vi "ATF-Obtain Notifier.vi"(8 "error in":errorcluster) -> (0 "error out":errorcluster, 3 "Cluster":T1)   [LabVIEW 2022 SP3]
uses:
  Controls/SeCrTs-Notifier ctl.ctl
  Controls/SeCrTs-NS Data type.ctl
  Controls/Commands to log.ctl
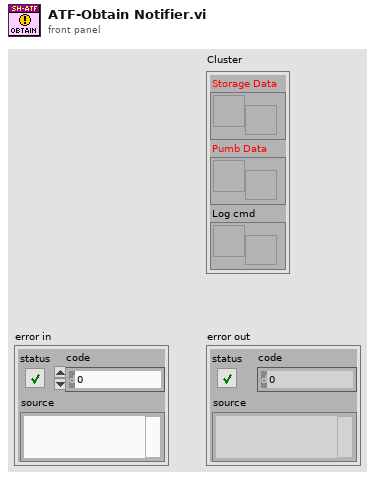
[diagram p1: front panel]
types:
  T1 = typedef "SeCrTs-Notifier ctl.ctl" = cluster{"Storage Data":refnum<notifier>, "Pumb Data":refnum<notifier>, "Log cmd":refnum<notifier>}
  T2 = typedef "Commands to log.ctl" = cluster{"C/NC":bool, "Start/Stop Log":bool[], "Log Name":string, "Config":cluster{"AO config":cluster{"Channel_Name":string, "Channel_Number":string, "Default_Value":dbl, "Units":string}[], "AI config":cluster{"Channel_Name":string, "Channel_Number":string, "Pre_Scale_min":dbl, "Pre_Scale_max":dbl, "Sensor_min":dbl, "Sensor_max":dbl, "Units":string}[], "DI config":cluster{"Channel_Name":string, "Channel_Number":string, "Default_Value":bool, "DI invert?":bool}[], "DO config":cluster{"Channel_Name":string, "Channel_Number":string, "Default_Value":bool, "DO invert?":bool}[], "TC config":cluster{"Channel_Name":string, "Channel_Number":string, "Pre_Scale_min":dbl, "Pre_Scale_max":dbl, "units":i32, " type":i32}[], "ACC config":cluster{"Channel_Name":string, "Channel_Number":string, "Pre_Scale_min":dbl, "Pre_Scale_max":dbl, "Terminal configuration":i32, "Sensitivity":dbl, "Sensitivity units":i32}[], "SG config":cluster{"Channel_Name":string, "Channel_Number":string, "Pre_Scale_min":dbl, "Pre_Scale_max":dbl}[], "Strain Gauge Settings":cluster{"poisson ratio":dbl, "nominal gage resistance":dbl, "gage factor":dbl}, "Bridge Settings":cluster{"voltage excitation value":dbl, "voltage excitation source":i32, "initial bridge voltage":dbl, "lead wire resistance":dbl, "strain configuration":i32}, "Sample Rate":cluster{"AI Sample Rate":dbl[], "AO Sample Rate":dbl[], "DI Sample Rate":dbl[], "TC Sample Rate":dbl[], "DO Sample Rate":dbl[], "SG Sample Rate":dbl[], "ACC Sample Rate":dbl[]}}, "Log min":dbl, "Drive":cluster{"Drive_Health":bool, "Drive_Frequency":u32, "Drive_Status":bool, "Drive_RPM":u32, "Drive_Direction":bool, "Acceleration state":bool, "Steady state":bool, "Deceleration state":bool, "Drive_Enable":bool, "Drive set_RPM":dbl}, "HOLD UPDATE":bool}
  T3 = typedef "SeCrTs-NS Data type.ctl" = cluster{"DI_Data":digitalwaveform[], "Drive_A_C":waveform(dbl)[], "Drive_A_D":waveform(dbl)[], "Drive_L_C":waveform(dbl)[], "Drive_L_D":waveform(dbl)[], "Loop Status":bool[], "CDT":dbl, "RT Error":cluster{"Error Code":string, "Error Source":string}, "DO":waveform(dbl)[], "SEQ Monitor":string[], "Device List":string}
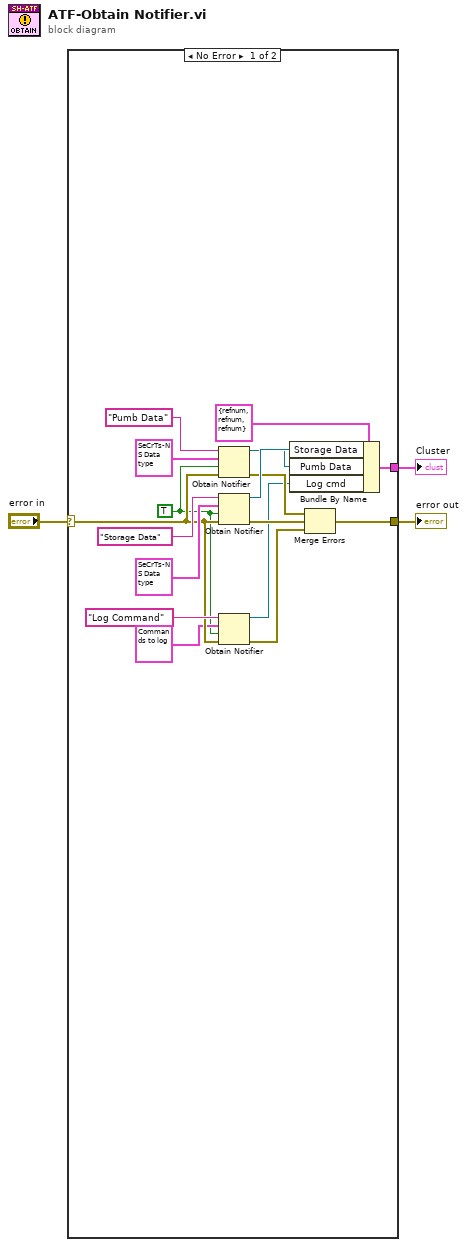
[diagram p0: block diagram]
diagram:
  n1 = case shown="No Error" "error in" {
    selector: "error in" -> [w8 w21]
    tunnel: [w10 w21] -> w2
    tunnel: [w18 _] -> w1
    frame No Error {
      w4 = TRUE ("create if not found? (T)")
      n2 = Obtain Notifier(name (unnamed)="Pumb Data", notification data type=T3 {"DI_Data"=[], "Drive_A_C"=[], "Drive_A_D"=[], "Drive_L_C"=[], "Drive_L_D"=[], "Loop Status"=[], "CDT"=0.0, "RT Error"={"Error Code"="", "Error Source"=""}, "DO"=[], "SEQ Monitor"=[], "Device List"=""} ("Read Data"), create if not found? (T)=w4, error in (no error)=w8) -> (notifier out=w13:refnum<notifier>, error out=w11:errorcluster)  [unwired: 1 out]
      n3 = Obtain Notifier(name (unnamed)="Storage Data", notification data type=T3 {"DI_Data"=[], "Drive_A_C"=[], "Drive_A_D"=[], "Drive_L_C"=[], "Drive_L_D"=[], "Loop Status"=[], "CDT"=0.0, "RT Error"={"Error Code"="", "Error Source"=""}, "DO"=[], "SEQ Monitor"=[], "Device List"=""} ("Read Data"), create if not found? (T)=w4, error in (no error)=w8) -> (notifier out=w16:refnum<notifier>, error out=w12:errorcluster)  [unwired: 1 out]
      n4 = Obtain Notifier(name (unnamed)="Log Command", notification data type=T2 {"C/NC"=FALSE, "Start/Stop Log"=[], "Log Name"="", "Config"={"AO config"=[], "AI config"=[], "DI config"=[], "DO config"=[], "TC config"=[], "ACC config"=[], "SG config"=[], "Strain Gauge Settings"={"poisson ratio"=0.0, "nominal gage resistance"=0.0, "gage factor"=0.0}, "Bridge Settings"={"voltage excitation value"=0.0, "voltage excitation source"=0, "initial bridge voltage"=0.0, "lead wire resistance"=0.0, "strain configuration"=0}, "Sample Rate"={"AI Sample Rate"=[], "AO Sample Rate"=[], "DI Sample Rate"=[], "TC Sample Rate"=[], "DO Sample Rate"=[], "SG Sample Rate"=[], "ACC Sample Rate"=[]}}, "Log min"=0.0, "Drive"={"Drive_Health"=FALSE, "Drive_Frequency"=0, "Drive_Status"=FALSE, "Drive_RPM"=0, "Drive_Direction"=FALSE, "Acceleration state"=FALSE, "Steady state"=FALSE, "Deceleration state"=FALSE, "Drive_Enable"=FALSE, "Drive set_RPM"=0.0}, "HOLD UPDATE"=FALSE} ("notification"), create if not found? (T)=w4, error in (no error)=w8) -> (notifier out=w5:refnum<notifier>, error out=w7:errorcluster)  [unwired: 1 out]
      n5 = Bundle By Name(cluster=T1 {"Storage Data"=refnum, "Pumb Data"=refnum, "Log cmd"=refnum} ("Cluster"), "Storage Data"=w16, "Pumb Data"=w13, "Log cmd"=w5) -> (w18:T1)
      n6 = Merge Errors(w11, w12, w7) -> (w10:errorcluster)
    }
    frame Error {
    }
  }
  "error out" <- w2
  "Cluster" <- w1
